vi "_PC_Pub getExeVersion.vi"(8 "error in (no error)":errorcluster) -> (0 "error out":errorcluster, 2 "path":string, 3 "version serial number":string)   [LabVIEW 2018]
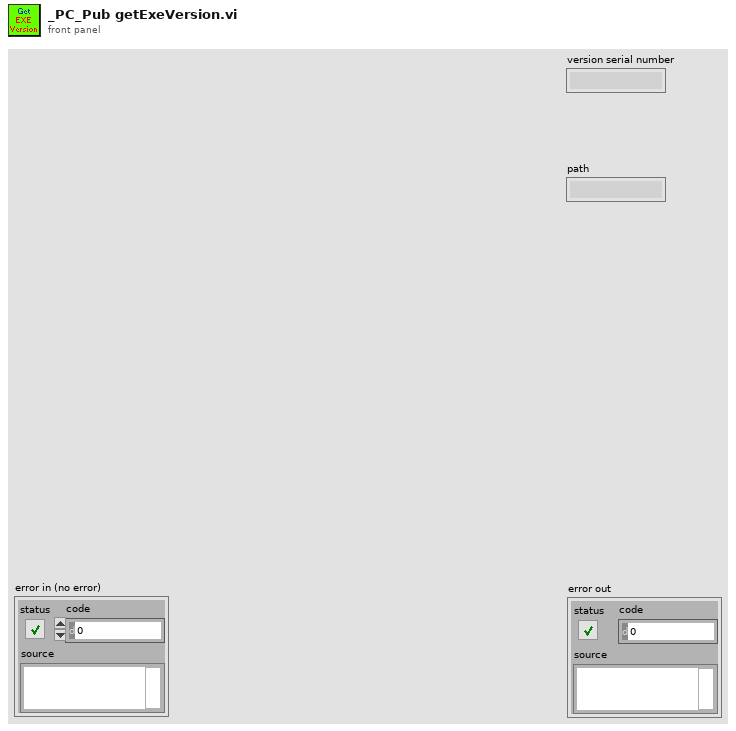
[diagram p1: front panel]
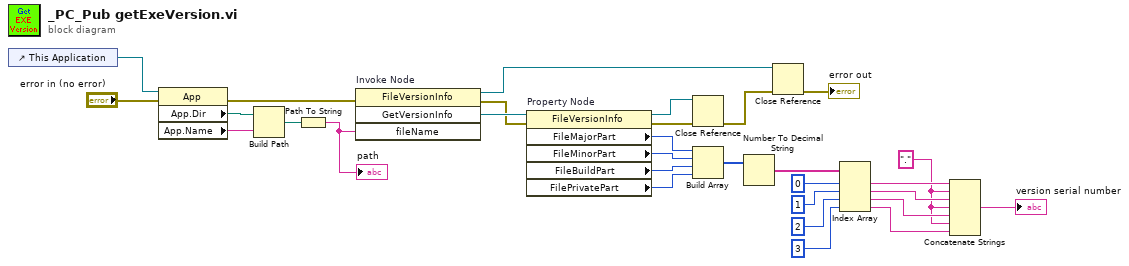
[diagram p0: block diagram]
diagram:
  w4 = "."
  n1 = control-ref of="This Application"() -> (w16:refnum<vi>)
  n2 = property class="App"(reference=w16, error in="error in (no error)") -> (error out=w1:errorcluster, "App.Dir"=w18:path, "App.Name"=w17:string)  [unwired: 1 out]
  n3 = Build Path(base path=w18, name or relative path=w17) -> (appended path=w15:path)
  n4 = Path To String(path=w15) -> (string=w30:string)
  "path" <- w30
  n5 = invoke on="Invoke Node" class="FileVersionInfo" method="GetVersionInfo"(error in=w1, "fileName"=w30) -> (reference out=w20:refnum<k24>, error out=w28:errorcluster, "GetVersionInfo"=w29:refnum<k24>)  [unwired: 2 in, 1 out]
  n6 = property on="Property Node" class="FileVersionInfo"(reference=w29, error in=w28) -> (reference out=w21:refnum<k24>, error out=w22:errorcluster, "FileMajorPart"=w27:i32, "FileMinorPart"=w26:i32, "FileBuildPart"=w25:i32, "FilePrivatePart"=w24:i32)
  n7 = Close Reference(reference=w21, error in (no error)=w22) -> (error out=w23:errorcluster)
  n8 = Build Array(w27, w26, w25, w24) -> (w14:i32[])
  n9 = Number To Decimal String(number=w14) -> (decimal integer string=w13:string[])  [unwired: 1 in]
  n10 = Close Reference(reference=w20, error in (no error)=w23) -> (error out=→"error out":errorcluster)
  n11 = Index Array(array=w13, index #1=0 ("index"), index #2=1 ("index"), index #3=2 ("index"), index #4=3 ("index")) -> (element #1=w8:string, element #2=w7:string, element #3=w6:string, element #4=w5:string)
  n12 = Concatenate Strings(w8, w4, w7, w4, w6, w4, w5) -> (→"version serial number":string)
